vi "Call-CryptoNight-Step-3-Fpga.vi"(8 "error in":errorcluster, 9 "Data in":u64[](array[numeric]) format="%.0x", 10 "Size-in":i32, 11 "Command":u32[](array[numeric]) format="%.0x") -> (0 "error out":errorcluster, 1 "b_out":u64[](array[numeric]) format="%.0x", 2 "a_out":u64[](array[numeric]) format="%.0x", 3 "Data out":u64[](array[numeric]))   [LabVIEW 2017]
uses:
  <vilib>/rvi/interface/RandomDataEmulation/nirviRandomDataOpen.vi
  <vilib>/rvi/interface/common/niFpgaCacheSessionInfoDynamic.vi
  <vilib>/Utility/error.llb/Error Cluster From Error Code.vi
  <vilib>/rvi/errors/niLvFpgaAdjustHostInterfaceError.vi
  <vilib>/FPGAPlugInAG/Dynamic/niLvFpga_Close_Dynamic.vi
  <vilib>/rvi/interface/nirviOpenFPGA/nirviOpenFPGA.xnode
  CryptoNight/FPGA/Fpga-Top-Level.vi
  <vilib>/rvi/interface/nirviReadWriteControl/nirviReadWriteControl.xnode
  <vilib>/rvi/interface/nirviMethod/nirviMethod.xnode
  <vilib>/rvi/interface/nirviCloseFPGA/nirviCloseFPGA.xnode
  NiFpgaLv.dll
  <vilib>/rvi/interface/Simulation/niFpgaSimulationCallBeginRW.vi
  <vilib>/FPGAPlugInAG/Dynamic/niLvFpga_WriteFifo_Dynamic.vi
  <vilib>/rvi/errors/niLvFpgaMergeErrorWithErrorCode.vi
  <vilib>/FPGAPlugInAG/Dynamic/niLvFpga_ReadFifo_Dynamic.vi
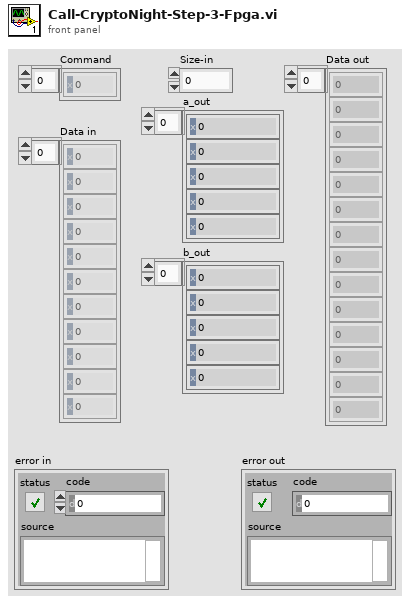
[diagram p1: front panel]
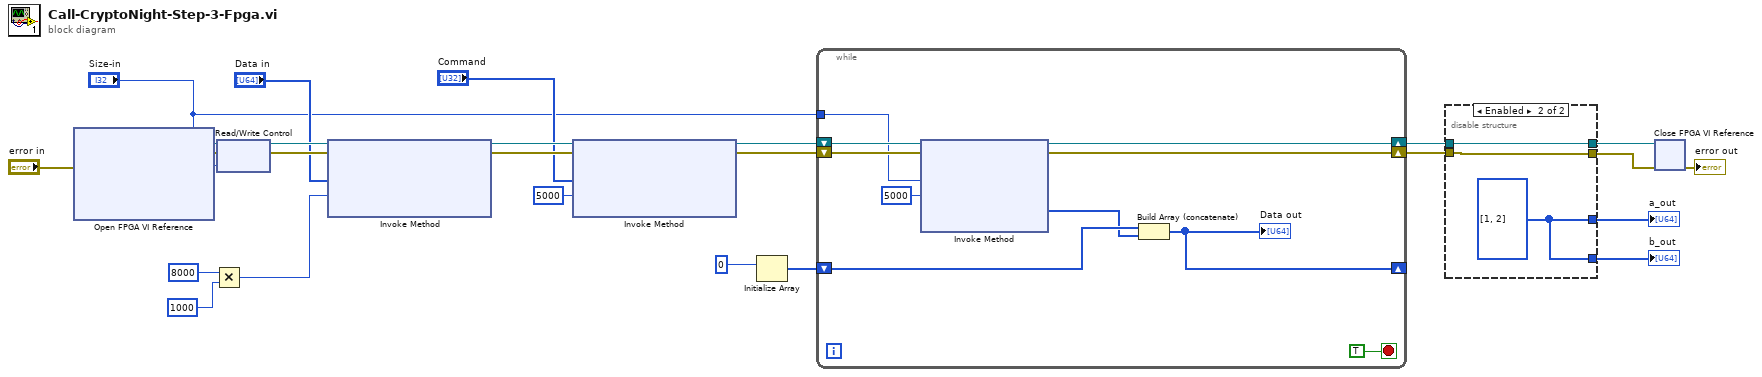
[diagram p0: block diagram]
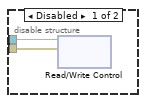
[diagram p2: hidden frame]
diagram:
  n1 = xnode "Open FPGA VI Reference"("error in"="error in") -> ("FPGA VI Reference Out"=w23:refnum<k20>, "error out"=w24:errorcluster)  [unwired: 1 in]
  n2 = Multiply(x=8000 ("Timeout (ms)"), y=1000 ("Timeout (ms)")) -> (x*y=w1:i32)
  n3 = xnode "Read/Write Control"("FPGA VI Reference In"=w23, "error in"=w24, "Size-in"="Size-in") -> ("FPGA VI Reference Out"=w22:refnum<k20>, "error out"=w21:errorcluster)
  n4 = xnode "Invoke Method"("FPGA VI Reference In"=w22, "error in"=w21, "Data"="Data in", "Timeout (ms)"=w1) -> ("FPGA VI Reference Out"=w19:refnum<k20>, "error out"=w18:errorcluster)  [unwired: 1 out]
  n5 = xnode "Invoke Method"("FPGA VI Reference In"=w19, "error in"=w18, "Data"="Command", "Timeout (ms)"=5000) -> ("FPGA VI Reference Out"=w15:refnum<k20>, "error out"=w14:errorcluster)  [unwired: 1 out]
  n6 = Initialize Array(u8 0) -> (w11:u8[])  [unwired: 1 in]
  n7 = while {
    shift-right: [w29] -> w8
    shift-left: w15 -> [w35]
    shift-right: [w28] -> w9
    shift-left: w14 -> [w34]
    tunnel: "Size-in" -> [w32]
    shift-right: [w27] -> _
    shift-left: w11 -> [w31]
    stop <- TRUE stop-if-true
    n8 = xnode "Invoke Method"("FPGA VI Reference In"=w35, "error in"=w34, "Number of Elements"=w32, "Timeout (ms)"=5000) -> ("FPGA VI Reference Out"=w29:refnum<k20>, "error out"=w28:errorcluster, "Data"=w30:u64[])  [unwired: 1 out]
    n9 = Build Array (concatenate)(w31, w30) -> (w27:u64[])
    "Data out" <- w27
  }
  n10 = disable-structure shown="Enabled" {
    disable-tunnel: w9 -> [w37 w39]
    disable-tunnel: w8 -> [w36 w40]
    disable-tunnel: [_ w40] -> w7
    disable-tunnel: [_ w39] -> w6
    disable-tunnel: [_ w38] -> w5
    disable-tunnel: [_ w38] -> w4
    frame Disabled {
      n11 = xnode "Read/Write Control"("FPGA VI Reference In"=w36, "error in"=w37) -> ()  [unwired: 1 in, 2 out]
    }
    frame Enabled {
      w38 = u64[] [1, 2] ("a_out")
    }
  }
  "a_out" <- w5
  "b_out" <- w4
  n12 = xnode "Close FPGA VI Reference"("FPGA VI Reference In"=w7, "error in"=w6) -> ("error out"=→"error out":errorcluster)
